vi "_nimcDMControlLoop_Multiply(32.16).vi"(2 "Gain":i16, 3 "Fraction":u16, 4 "Integer":i32) -> (0 "Fraction":u16, 1 "Integer":i32)   [LabVIEW 2014]
doc: "Performs fixed point multiplication. X operand is in 32.16 format, Y operand is in 16.0 format and result is in 32.16 format."
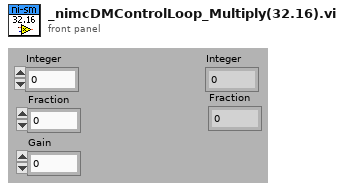
[diagram p1: front panel]
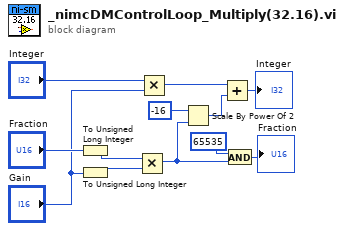
[diagram p0: block diagram]
diagram:
  n1 = To Unsigned Long Integer(number="Fraction") -> (unsigned 32bit integer=w2:u32)
  n2 = To Unsigned Long Integer(number="Gain") -> (unsigned 32bit integer=w1:u32)
  n3 = Multiply(x=w2, y=w1) -> (x*y=w3:u32)
  n4 = Multiply(x="Integer", y="Gain") -> (x*y=w4:i32)
  n5 = Scale By Power Of 2(n=i16 -16, x=w3) -> (x*2^n=w7:u32)
  n6 = Add(x=w4, y=w7) -> (x+y=→"Integer":u32)
  n7 = And(x=65535, y=w3) -> (x .and. y?=→"Fraction":u32)
